vi "ImportBehFile.vi"(8 "error in (no error)":errorcluster, 9 "reference":refnum<vi>, 10 "beh_file":T1, 11 "Database in":refnum<class "Database.lvclass">) -> (0 "error out":errorcluster, 1 "reference 2":refnum<vi>, 3 "Database out":refnum<class "Database.lvclass">)   [LabVIEW 2014, in "Database.lvclass"]
uses:
  Database.lvclass
  Database.lvclass/Database.ctl
  <vilib>/addons/database/NI_Database_API.lvlib
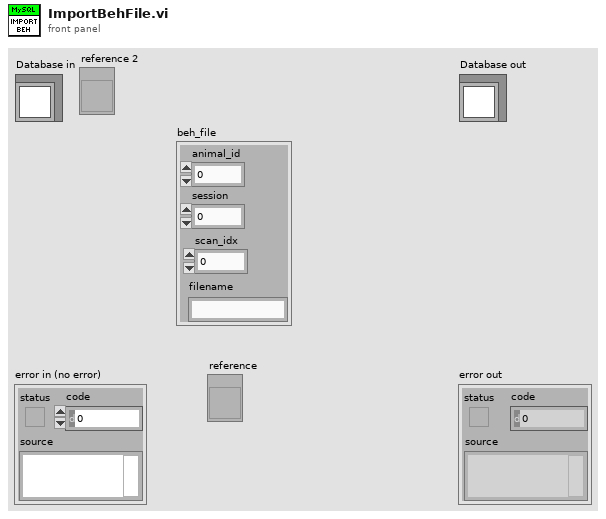
[diagram p1: front panel]
types:
  T1 = cluster{"animal_id":dbl, "session":dbl, "scan_idx":dbl, "filename":string}
  T2 = typedef "NI_Database_API.lvlib/Conn ObjectReference.ctl" = refnum<k1>
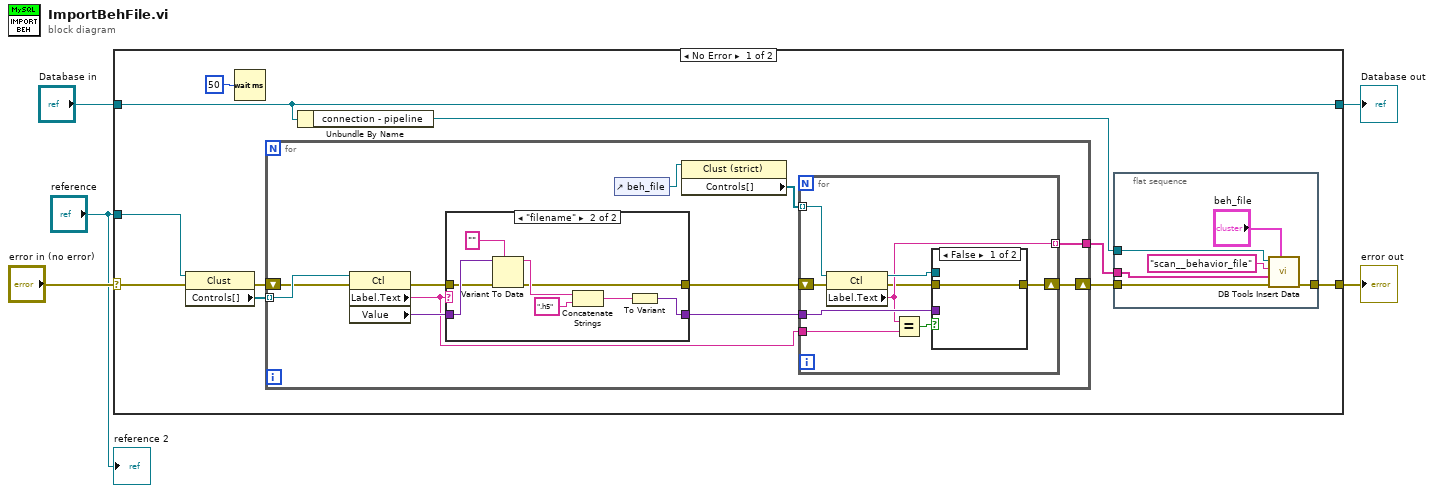
[diagram p0: block diagram]
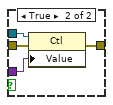
[diagram p3: hidden frame]
diagram:
  n1 = case shown="No Error" "error in (no error)" {
    selector: "error in (no error)" -> [w9 w58]
    tunnel: [w7 w58] -> w2
    tunnel: [w8 w57] -> w3
    tunnel: "Database in" -> [w8 w57]
    tunnel: "reference" -> [w6 _]
    frame No Error {
      n2 = property class="Clust"(reference=w6, error in=w9) -> (error out=w14:errorcluster, "Controls[]"=w15:refnum<vi>[])  [unwired: 1 out]
      n3 = Wait (ms)(milliseconds to wait=u32 50) -> ()  [unwired: 1 out]
      n4 = for {
        tunnel: w15 -> [w32] mode=indexing
        shift-right: [w23] -> w11
        shift-left: w14 -> [w31]
        tunnel: [w29] -> w13
        n5 = property class="Ctl"(reference=w32, error in=w31) -> (error out=w27:errorcluster, "Label.Text"=w22:string, "Value"=w25:variant)  [unwired: 1 out]
        n6 = case shown="\"filename\"" w22 {
          tunnel: w27 -> [w33 w35]
          tunnel: w25 -> [w34 w42]
          tunnel: [w34 w41] -> w24
          tunnel: [w33 w36] -> w26
          frame "False", Default {
          }
          frame "filename" {
            n7 = Variant To Data(error in=w35, type="", Variant=w42) -> (data=w39:string, error out=w36:errorcluster)
            n8 = Concatenate Strings(w39, ".h5" ("string")) -> (w37:string)
            n9 = To Variant(anything=w37) -> (Variant=w41:variant)
          }
        }
        n10 = control-ref of="beh_file"() -> (w30:refnum<vi>)
        n11 = property class="Clust (strict)"(reference=w30) -> ("Controls[]"=w28:refnum<vi>[])  [unwired: 1 in, 2 out]
        n12 = for {
          tunnel: w22 -> [w51]
          tunnel: w24 -> [w48]
          tunnel: w28 -> [w50] mode=indexing
          tunnel: [w46] -> w29 mode=indexing
          shift-right: [w44] -> w23
          shift-left: w26 -> [w43]
          n13 = property class="Ctl"(reference=w50, error in=w43) -> (reference out=w49:refnum<vi>, error out=w45:errorcluster, "Label.Text"=w46:string)
          n14 = Equal?(x=w46, y=w51) -> (x = y?=w47:bool)
          n15 = case shown="False" w47 {
            tunnel: w49 -> [_ w56]
            tunnel: w48 -> [_ w55]
            tunnel: w45 -> [w52 w54]
            tunnel: [w52 w53] -> w44
            frame False {
            }
            frame True {
              n16 = property class="Ctl"(reference=w56, error in=w54, "Value"=w55) -> (error out=w53:errorcluster)  [unwired: 1 out]
            }
          }
        }
      }
      n17 = Unbundle By Name(w8) -> ("connection - pipeline"=w12:T2)
      n18 = flat-sequence {
        tunnel: w13 -> [w21]
        tunnel: w12 -> [w20]
        tunnel: w11 -> [w19]
        tunnel: [w17] -> w7
        frame #0 {
          n19 = call <vilib>:"DB Tools Insert Data.vi"("data"="beh_file", "error in (no error)"=w19, "columns"=w21, "table"="scan__behavior_file" ("session"), "connection reference"=w20) -> ("error out"=w17:errorcluster)  [unwired: 5 in, 1 out]
        }
      }
    }
    frame Error {
    }
  }
  "error out" <- w2
  "Database out" <- w3
  "reference 2" <- "reference"
